vi "Alphabetize.vi"(8 "Error In":errorcluster, 11 "Clusters In":refnum<vi>[](array[refnum])) -> (0 "Error Out":errorcluster, 2 "Change?":bool, 3 "Clusters Out":refnum<vi>[](array[refnum]))   [LabVIEW 2017, in "Toolkit.lvlib"]
doc: "Alphabetizes all elements in all clusters. If the GObject reference is not to a cluster constant or control, then it is silently skipped. Only clusters will be alphabetized."
uses:
  Toolkit.lvlib
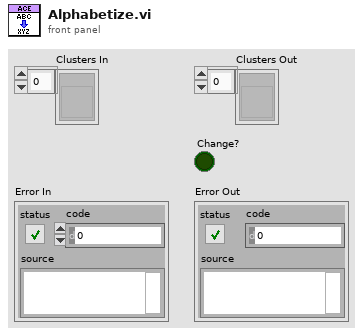
[diagram p1: front panel]
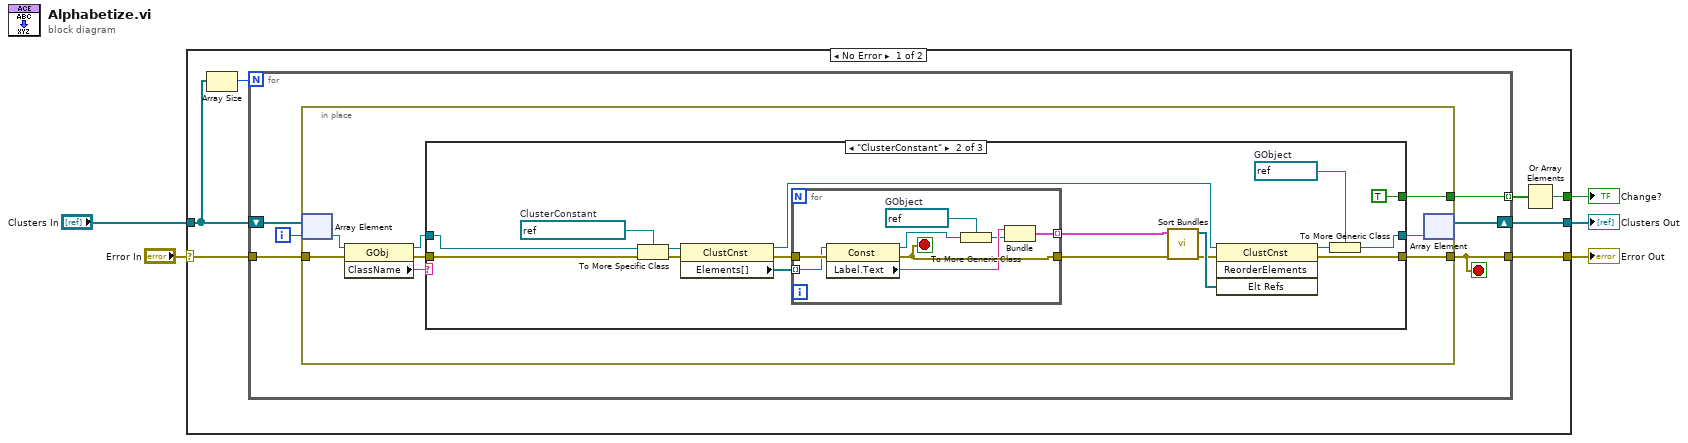
[diagram p0: block diagram]
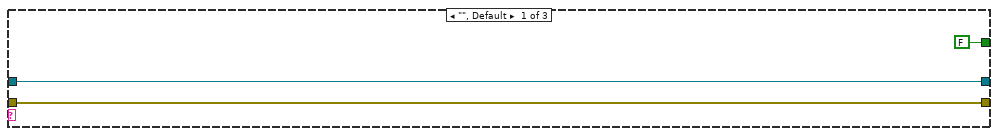
[diagram p2: hidden frame]
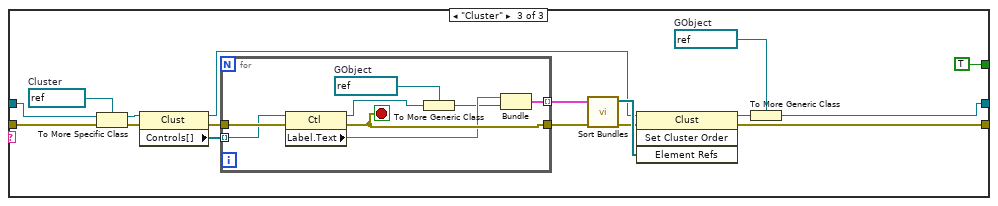
[diagram p3: hidden frame]
diagram:
  n1 = case shown="No Error" "Error In" {
    selector: "Error In" -> [w12 w81]
    tunnel: [w11 w81] -> w4
    tunnel: "Clusters In" -> [w9 w80]
    tunnel: [w10 w80] -> w2
    tunnel: [w6 _] -> w1
    frame No Error {
      n2 = Array Size(array=w9) -> (size(s)=w8:i32)
      n3 = for {
        N: w8 -> [_]
        tunnel: w12 -> [w18]
        tunnel: [w14] -> w11
        shift-right: [w15] -> w10
        shift-left: w9 -> [w17]
        tunnel: [w13] -> w7 mode=indexing
        i -> [w16]
        stop <- w14 stop-if-true
        n4 = in-place {
          in-place-border: w18 -> [w25]
          in-place-border: [w21] -> w14
          in-place-border: [w19] -> w13
          n5 = in-place-array #1(w17, w16) -> (w26:refnum<vi>)
          n6 = property class="GObj"(reference=w26, error in=w25) -> (reference out=w22:refnum<vi>, error out=w23:errorcluster, "ClassName"=w24:string)
          n7 = case shown="\"ClusterConstant\"" w24 {
            tunnel: w23 -> [w28 w46 w71]
            tunnel: w22 -> [w29 w45 w70]
            tunnel: [w28 w34 w59] -> w21
            tunnel: [w29 w31 w56] -> w20
            tunnel: [FALSE TRUE TRUE] -> w19
            frame "", Default {
            }
            frame "ClusterConstant" {
              w33 = refnum<vi> refnum  # GObject
              w44 = refnum<vi> refnum  # ClusterConstant
              n8 = To More Specific Class(target class=w44, reference=w45, error in=w46) -> (specific class reference=w43:refnum<vi>, error out=w42:errorcluster)
              n9 = property class="ClustCnst"(reference=w43, error in=w42) -> (reference out=w37:refnum<vi>, error out=w36:errorcluster, "Elements[]"=w35:refnum<vi>[])
              n10 = for {
                tunnel: w36 -> [w54]
                tunnel: [w53] -> w39
                tunnel: w35 -> [w50] mode=indexing
                tunnel: [w51] -> w38 mode=indexing
                stop <- w53 stop-if-true
                w48 = refnum<vi> refnum  # GObject
                n11 = property class="Const"(reference=w50, error in=w54) -> (reference out=w49:refnum<vi>, error out=w53:errorcluster, "Label.Text"=w52:string)
                n12 = To More Generic Class(target class=w48, reference=w49) -> (generic class reference=w47:refnum<vi>)
                n13 = Bundle("Label.Text"=w52, w47) -> (w51:cluster{"Label.Text":string, refnum<vi>})  [unwired: 1 in]
              }
              n14 = call "Sort Bundles.vi"("Error In"=w39, "Bundles"=w38) -> ("Error Out"=w40:errorcluster, "Sorted Elements"=w41:refnum<vi>[])  [unwired: 8 in]
              n15 = invoke class="ClustCnst" method="ReorderElements"(reference=w37, error in=w40, "Elt Refs"=w41) -> (reference out=w32:refnum<vi>, error out=w34:errorcluster)  [unwired: 1 in, 2 out]
              n16 = To More Generic Class(target class=w33, reference=w32) -> (generic class reference=w31:refnum<vi>)
            }
            frame "Cluster" {
              w57 = refnum<vi> refnum  # GObject
              w69 = refnum<vi> refnum  # Cluster
              n17 = To More Specific Class(target class=w69, reference=w70, error in=w71) -> (specific class reference=w68:refnum<vi>, error out=w67:errorcluster)
              n18 = property class="Clust"(reference=w68, error in=w67) -> (reference out=w62:refnum<vi>, error out=w61:errorcluster, "Controls[]"=w60:refnum<vi>[])
              n19 = for {
                tunnel: w61 -> [w79]
                tunnel: [w78] -> w64
                tunnel: w60 -> [w75] mode=indexing
                tunnel: [w76] -> w63 mode=indexing
                stop <- w78 stop-if-true
                w73 = refnum<vi> refnum  # GObject
                n20 = property class="Ctl"(reference=w75, error in=w79) -> (reference out=w74:refnum<vi>, error out=w78:errorcluster, "Label.Text"=w77:string)
                n21 = To More Generic Class(target class=w73, reference=w74) -> (generic class reference=w72:refnum<vi>)
                n22 = Bundle("Label.Text"=w77, w72) -> (w76:cluster{"Label.Text":string, refnum<vi>})  [unwired: 1 in]
              }
              n23 = call "Sort Bundles.vi"("Error In"=w64, "Bundles"=w63) -> ("Error Out"=w65:errorcluster, "Sorted Elements"=w66:refnum<vi>[])  [unwired: 8 in]
              n24 = invoke class="Clust" method="Set Cluster Order"(reference=w62, error in=w65, "Element Refs"=w66) -> (reference out=w58:refnum<vi>, error out=w59:errorcluster)  [unwired: 1 in, 2 out]
              n25 = To More Generic Class(target class=w57, reference=w58) -> (generic class reference=w56:refnum<vi>)
            }
          }
          n26 = in-place-array #1(w20) -> (w15:refnum<vi>[])  [unwired: 1 out]
        }
      }
      n27 = Or Array Elements(Boolean array=w7) -> (logical OR=w6:bool)
    }
    frame Error {
    }
  }
  "Error Out" <- w4
  "Clusters Out" <- w2
  "Change?" <- w1
